vi "TestPaths.vi"() -> ()   [LabVIEW 2018]
panel:
  out "Click the starting location/loading station, then the desired scoring destination":T1(plugin-control)
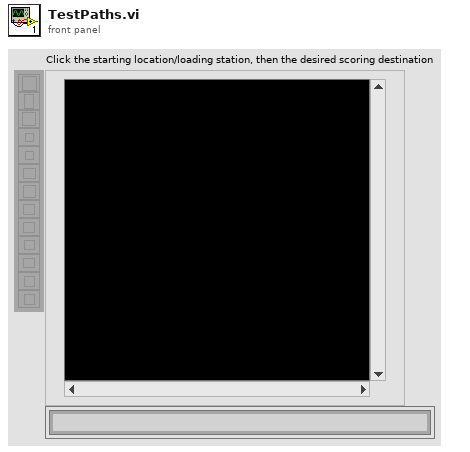
[diagram p1: front panel]
types:
  T1 = typedef "IMAQ Image.ctl" = refnum<image>
  T2 = typedef "Image Type" = u32
  T3 = typedef "LVPoint32TypeDef.ctl" = cluster{"Horizontal":i32, "Vertical":i32}
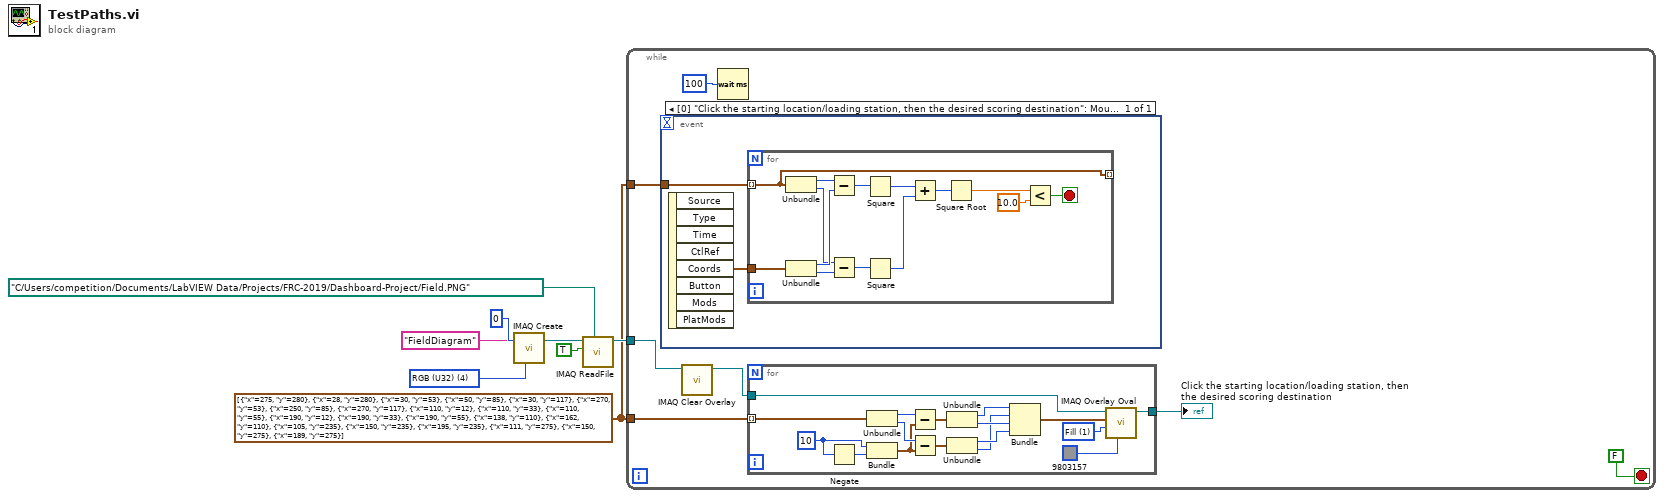
[diagram p0: block diagram]
diagram:
  w1 = cluster{"x":i32, "y":i32}[] [{"x"=275, "y"=280}, {"x"=28, "y"=280}, {"x"=30, "y"=53}, {"x"=50, "y"=85}, {"x"=30, "y"=117}, {"x"=270, "y"=53}, {"x"=250, "y"=85}, {"x"=270, "y"=117}, {"x"=110, "y"=12}, {"x"=110, "y"=33}, {"x"=110, "y"=55}, {"x"=190, "y"=12}, {"x"=190, "y"=33}, {"x"=190, "y"=55}, {"x"=138, "y"=110}, {"x"=162, "y"=110}, {"x"=105, "y"=235}, {"x"=150, "y"=235}, {"x"=195, "y"=235}, {"x"=111, "y"=275}, {"x"=150, "y"=275}, {"x"=189, "y"=275}]
  w6 = T2 4 items=["Grayscale (U8)", "Grayscale (I16)", "Grayscale (SGL)", "Complex (CSG)", "RGB (U32)", "HSL (U32)", "RGB (U64)", "Grayscale (U16)"] ("Image Type")
  n1 = call "IMAQ Create"("Border Size"=0, "Image Name"="FieldDiagram", "Image Type"=w6) -> ("New Image"=w5:T1)  [unwired: 2 in, 1 out]
  n2 = call "IMAQ ReadFile"("File Path"=path "C:/Users/competition/Documents/LabVIEW Data/Projects/FRC-2019/Dashboard-Project/Field.PNG", "Load Color Palette? (No)"=TRUE, "Image"=w5) -> ("Image Out"=w2:T1)  [unwired: 4 in, 4 out]
  n3 = while {
    tunnel: w2 -> [w11]
    tunnel: w1 -> [w13]
    tunnel: w1 -> [w9]
    stop <- FALSE stop-if-true
    n4 = event shown="[0] \"Click the starting location/loading station, then the desired scoring destination\": Mouse Down" {
      selector: _ -> [_]
      dyn-events: _ -> [_]
      timeout: _ -> [_]
      tunnel: w9 -> [w17]
      event "Click the starting location/loading station, then the desired scoring destination": Mouse Down {
        n5 = event-data() -> ("Coords"=w16:T3)  [unwired: 1 in, 7 out]
        n6 = for {
          tunnel: w17 -> [w18] mode=indexing
          tunnel: w16 -> [w31]
          tunnel: [w18] -> _ mode=indexing
          stop <- w19 stop-if-true
          n7 = Unbundle(w18) -> ("x"=w30:i32, "y"=w27:i32)
          n8 = Unbundle(w31) -> ("Horizontal"=w29:i32, "Vertical"=w28:i32)
          n9 = Subtract(x=w30, y=w29) -> (x-y=w26:i32)
          n10 = Subtract(x=w27, y=w28) -> (x-y=w25:i32)
          n11 = Square(x=w26) -> (x^2=w24:i32)
          n12 = Square(x=w25) -> (x^2=w20:i32)
          n13 = Add(x=w24, y=w20) -> (x+y=w23:i32)
          n14 = Square Root(x=w23) -> (sqrt(x)=w22:dbl)
          n15 = Less?(x=w22, y=10.0) -> (x < y?=w19:bool)
        }
      }
    }
    n16 = call "IMAQ Clear Overlay"("Image"=w11) -> ("Image Out"=w10:T1)  [unwired: 9 in, 1 out]
    n17 = Wait (ms)(milliseconds to wait=u32 100) -> ()  [unwired: 1 out]
    n18 = for {
      tunnel: w13 -> [w48] mode=indexing
      tunnel: w10 -> [w42]
      tunnel: [w41] -> w12
      w33 = u32 1 items=["Frame", "Fill"] ("Drawing Mode (Frame)")
      w39 = 10
      n19 = Negate(x=w39) -> (-x=w38:i32)
      n20 = Unbundle(w48) -> ("x"=w47:i32, "y"=w43:i32)
      n21 = Bundle(w39, w38) -> (w40:cluster{i32, i32})  [unwired: 1 in]
      n22 = Subtract(x=w47, y=w40) -> (x-y=w45:cluster{i32, i32})
      n23 = Subtract(x=w43, y=w40) -> (x-y=w44:cluster{i32, i32})
      n24 = Unbundle(w45) -> (w46:i32, w37:i32)
      n25 = Unbundle(w44) -> (w36:i32, w35:i32)
      n26 = Bundle(w46, w35, w37, w36) -> (w32:cluster{i32, i32, i32, i32})  [unwired: 1 in]
      n27 = call "IMAQ Overlay Oval"("Color"=u32 9803157, "Drawing Mode (Frame)"=w33, "Bounding Rectangle"=w32, "Image"=w42) -> ("Image Out"=w41:T1)  [unwired: 6 in, 1 out]
    }
    "Click the starting location/loading station, then the desired scoring destination" <- w12
  }
